vi "TCPReadVariable.vi"(7 "String Var?":bool, 8 "error in (no error)":errorcluster, 9 "timeout ms (25000)":i32, 10 "command":string, 11 "connection ID":refnum<k5>) -> (0 "error out":errorcluster, 2 "Variable":T1, 3 "connection ID out":refnum<k5>)   [LabVIEW 2013]
uses:
  FBVar.ctl
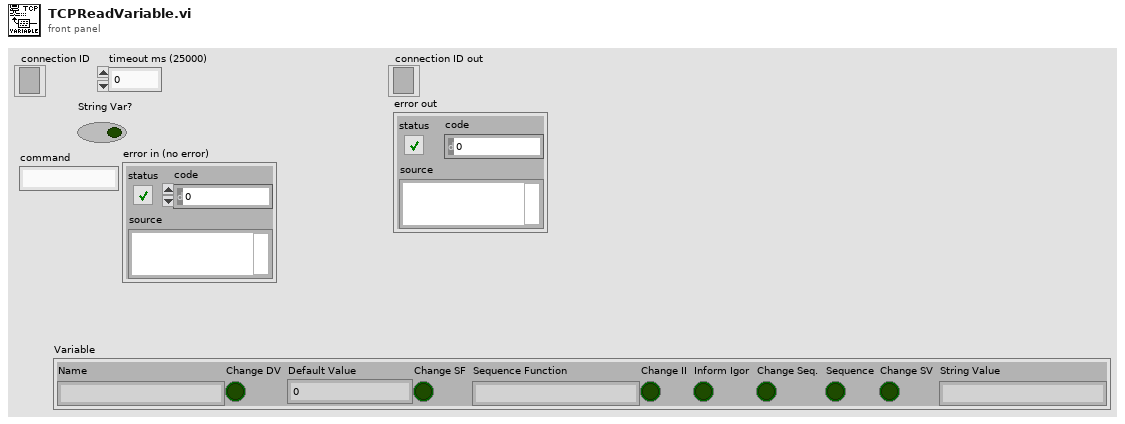
[diagram p1: front panel]
types:
  T1 = typedef "FBVar.ctl" = cluster{"Name":string, "Change DV":bool, "Default Value":dbl, "Change SF":bool, "Sequence Function":string, "Change II":bool, "Inform Igor":bool, "Change Seq.":bool, "Sequence":bool, "Change SV":bool, "String Value":string}
  T2 = cluster{"Boolean array[0]":bool, "Boolean array[1]":bool, "Boolean array[2]":bool, "Boolean array[3]":bool, "Boolean array[4]":bool, "Boolean array[5]":bool, "Boolean array[6]":bool, "Boolean array[7]":bool}
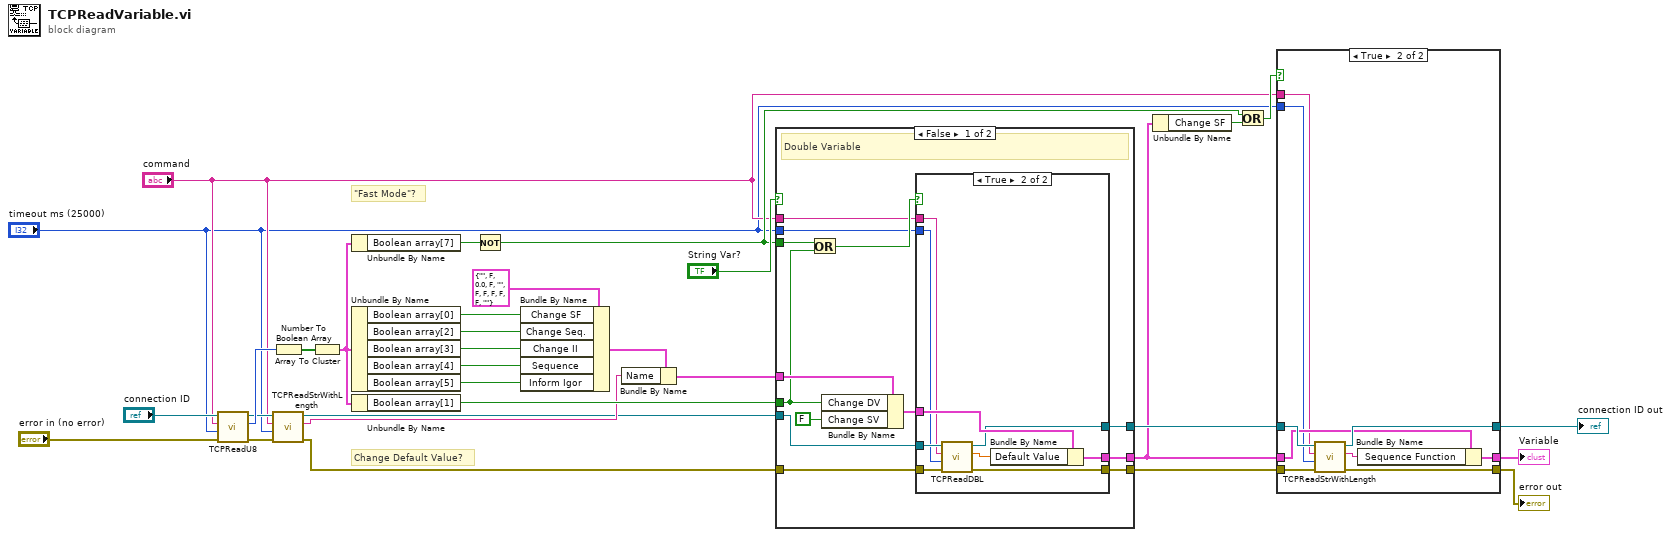
[diagram p0: block diagram]
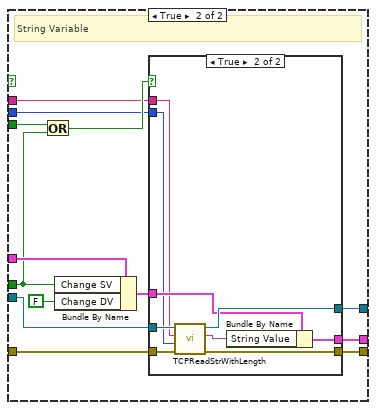
[diagram p4: hidden frame]
diagram:
  # "\"Fast Mode\"?"
  # "Change Default Value?"
  n1 = call "TCPReadU8.vi"("error in (no error)"="error in (no error)", "timeout ms (25000)"="timeout ms (25000)", "command"="command", "connection ID"="connection ID") -> ("error out"=w31:errorcluster, "U8 value"=w32:u8, "connection ID out"=w30:refnum<k5>)  [unwired: 5 in]
  n2 = call "TCPReadStrWithLength.vi"("error in (no error)"=w31, "timeout ms (25000)"="timeout ms (25000)", "command"="command", "connection ID"=w30) -> ("error out"=w17:errorcluster, "TCP String"=w20:string, "connection ID out"=w16:refnum<k5>)  [unwired: 5 in]
  n3 = Number To Boolean Array(number=w32) -> (Boolean array=w29:bool[])
  n4 = Array To Cluster(array=w29) -> (cluster=w19:T2)
  n5 = Unbundle By Name(w19) -> ("Boolean array[7]"=w18:bool)
  n6 = Unbundle By Name(w19) -> ("Boolean array[0]"=w28:bool, "Boolean array[2]"=w27:bool, "Boolean array[3]"=w26:bool, "Boolean array[4]"=w25:bool, "Boolean array[5]"=w24:bool)
  n7 = Unbundle By Name(w19) -> ("Boolean array[1]"=w22:bool)
  n8 = Not(x=w18) -> (.not. x?=w13:bool)
  n9 = Bundle By Name(cluster=T1 {"Name"="", "Change DV"=FALSE, "Default Value"=0.0, "Change SF"=FALSE, "Sequence Function"="", "Change II"=FALSE, "Inform Igor"=FALSE, "Change Seq."=FALSE, "Sequence"=FALSE, "Change SV"=FALSE, "String Value"=""} ("Variable"), "Change SF"=w28, "Change Seq."=w27, "Change II"=w26, "Sequence"=w25, "Inform Igor"=w24) -> (w15:T1)
  n10 = Bundle By Name(cluster=w15, "Name"=w20) -> (w14:T1)
  n11 = case shown="False" "String Var?" {
    tunnel: w22 -> [w42 w65]
    tunnel: w14 -> [w45 w70]
    tunnel: w17 -> [w38 w68]
    tunnel: w16 -> [w37 w67]
    tunnel: w13 -> [w43 w66]
    tunnel: [w36 w63] -> w10
    tunnel: [w39 w62] -> w9
    tunnel: [w40 w60] -> w8
    tunnel: "command" -> [w34 w59]
    tunnel: "timeout ms (25000)" -> [w33 w58]
    frame False {
      # "Double Variable"
      n12 = Or(x=w43, y=w42) -> (x .or. y?=w35:bool)
      n13 = Bundle By Name(cluster=w45, "Change DV"=w42, "Change SV"=FALSE) -> (w41:T1)
      n14 = case shown="True" w35 {
        tunnel: w41 -> [w46 w57]
        tunnel: [w46 w56] -> w40
        tunnel: [w48 w54] -> w39
        tunnel: w38 -> [w48 w53]
        tunnel: w37 -> [w47 w52]
        tunnel: [w47 w51] -> w36
        tunnel: w34 -> [_ w50]
        tunnel: w33 -> [_ w49]
        frame False {
        }
        frame True {
          n15 = call "TCPReadDBL.vi"("error in (no error)"=w53, "timeout ms (25000)"=w49, "command"=w50, "connection ID"=w52) -> ("error out"=w54:errorcluster, "DBL value"=w55:dbl, "connection ID out"=w51:refnum<k5>)  [unwired: 5 in]
          n16 = Bundle By Name(cluster=w57, "Default Value"=w55) -> (w56:T1)
        }
      }
    }
    frame True {
      # "String Variable"
      n17 = Or(x=w66, y=w65) -> (x .or. y?=w64:bool)
      n18 = Bundle By Name(cluster=w70, "Change SV"=w65, "Change DV"=FALSE) -> (w61:T1)
      n19 = case shown="True" w64 {
        tunnel: w68 -> [w71 w82]
        tunnel: w67 -> [w72 w81]
        tunnel: [w72 w80] -> w63
        tunnel: [w71 w79] -> w62
        tunnel: w61 -> [w73 w78]
        tunnel: [w73 w76] -> w60
        tunnel: w59 -> [_ w75]
        tunnel: w58 -> [_ w74]
        frame False {
        }
        frame True {
          n20 = call "TCPReadStrWithLength.vi"("error in (no error)"=w82, "timeout ms (25000)"=w74, "command"=w75, "connection ID"=w81) -> ("error out"=w79:errorcluster, "TCP String"=w77:string, "connection ID out"=w80:refnum<k5>)  [unwired: 5 in]
          n21 = Bundle By Name(cluster=w78, "String Value"=w77) -> (w76:T1)
        }
      }
    }
  }
  n22 = Unbundle By Name(w8) -> ("Change SF"=w12:bool)
  n23 = Or(x=w13, y=w12) -> (x .or. y?=w11:bool)
  n24 = case shown="True" w11 {
    tunnel: w10 -> [w85 w93]
    tunnel: w9 -> [w84 w94]
    tunnel: [w85 w92] -> w3
    tunnel: [w84 w91] -> w2
    tunnel: w8 -> [w83 w90]
    tunnel: [w83 w89] -> w1
    tunnel: "command" -> [_ w87]
    tunnel: "timeout ms (25000)" -> [_ w86]
    frame False {
    }
    frame True {
      n25 = call "TCPReadStrWithLength.vi"("error in (no error)"=w94, "timeout ms (25000)"=w86, "command"=w87, "connection ID"=w93) -> ("error out"=w91:errorcluster, "TCP String"=w88:string, "connection ID out"=w92:refnum<k5>)  [unwired: 5 in]
      n26 = Bundle By Name(cluster=w90, "Sequence Function"=w88) -> (w89:T1)
    }
  }
  "connection ID out" <- w3
  "error out" <- w2
  "Variable" <- w1
